vi "Configure Modulation (Pulse Width).vi"(0 "VISA resource name":refnum<visa-resource-name>, 1 "PWM Source (0: Internal)":i32(ring) items=["Internal", "External", "CH1", "CH2"], 2 "Internal Function (0: Sine)":i32(ring) items=["Sine", "Square", "RAMP", "NRAMP", "Triangle", "Noise", "PRBS", "Arbitrary"], 3 "PWM Deviation Duty Cycle (1 Percent)":dbl=1.0, 5 "Channel (1: 1)":i32(ring)=1 items=["1"=1, "2"=2], 7 "Enable Pulse Width Modulation(T: Enable)":bool=TRUE, 11 "error in (no error)":errorcluster, 12 "Deviation Setting Mode (0: Normal)":i32(ring) items=["Normal", "Duty Cycle"], 13 "PWM Internal Frequency/Sample Rate (10 Hz)":dbl=10.0, 14 "PWM Deviation (10 us)":dbl=1e-05) -> (4 "VISA resource name out":refnum<visa-resource-name>, 15 "error out":errorcluster)   [LabVIEW 2015, in "Agilent 3352X Series.lvlib"]
doc: "Allows and configures pulse width modulation. The width of a pulse waveform is varied by the instantaneous voltage of the modulating waveform.\n\n<b>Note</b>:\n(1) Before using this mode, all other modes must be turned off.\n(2) The carrier waveform must be Pulse.\n(3) The carrier waveform parameters are set by the Configure Pulse Waveform.vi"
uses:
  <instrlib>/Agilent 3352X Series/Agilent 3352X Series.lvlib
panel:
  # "Internal Pulse Width Modulation Settings"
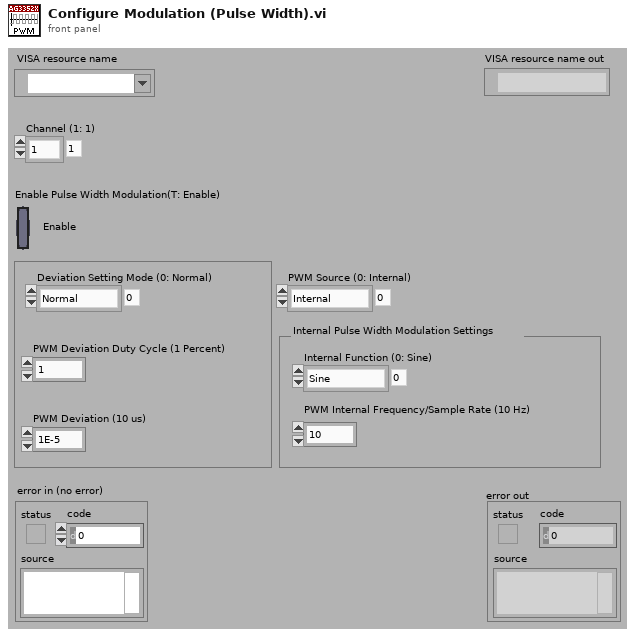
[diagram p1: front panel]
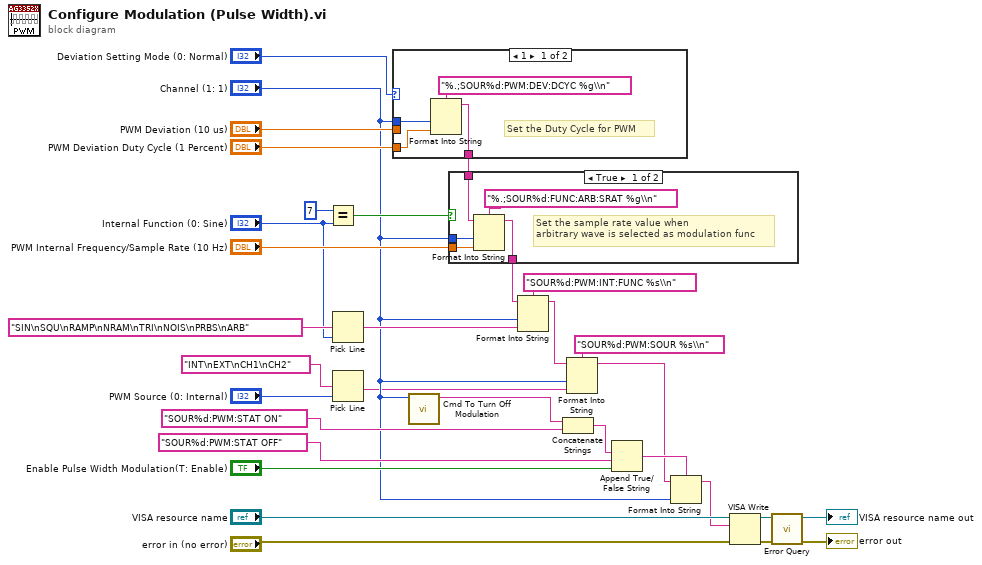
[diagram p0: block diagram]
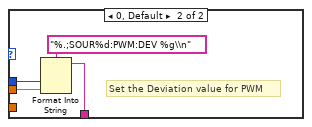
[diagram p2: hidden frame]
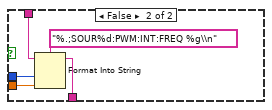
[diagram p3: hidden frame]
diagram:
  n1 = Equal?(x=u16 7, y="Internal Function (0: Sine)") -> (x = y?=w15:bool)
  n2 = Pick Line(multi-line string="SIN\nSQU\nRAMP\nNRAM\nTRI\nNOIS\nPRBS\nARB", line index="Internal Function (0: Sine)") -> (output string=w21:string)  [unwired: 1 out]
  n3 = Pick Line(multi-line string="INT\nEXT\nCH1\nCH2", line index="PWM Source (0: Internal)") -> (output string=w1:string)  [unwired: 1 out]
  n4 = case shown="1" "Deviation Setting Mode (0: Normal)" {
    tunnel: "Channel (1: 1)" -> [w35 w39]
    tunnel: "PWM Deviation (10 us)" -> [_ w38]
    tunnel: "PWM Deviation Duty Cycle (1 Percent)" -> [w34 _]
    tunnel: [w33 w37] -> w12
    frame 1 {
      # "Set the Duty Cycle for PWM"
      n5 = Format Into String(format string="%.;SOUR%d:PWM:DEV:DCYC %g\\n", w35, w34) -> (resulting string=w33:string)  [unwired: 2 in, 1 out]
    }
    frame 0, Default {
      # "Set the Deviation value for PWM"
      n6 = Format Into String(format string="%.;SOUR%d:PWM:DEV %g\\n", w39, w38) -> (resulting string=w37:string)  [unwired: 2 in, 1 out]
    }
  }
  n7 = call <instrlib>:"Cmd To Turn Off Modulation.vi"("Channel (1: 1)"="Channel (1: 1)") -> ("Cmd String"=w7:string)  [unwired: 10 out]
  n8 = case shown="True" w15 {
    tunnel: "Channel (1: 1)" -> [w43 w50]
    tunnel: w12 -> [w41 w49]
    tunnel: "PWM Internal Frequency/Sample Rate (10 Hz)" -> [w42 w47]
    tunnel: [w45 w46] -> w18
    frame True {
      # "Set the sample rate value when\narbitrary wave is selected as modulation func"
      n9 = Format Into String(format string="%.;SOUR%d:FUNC:ARB:SRAT %g\\n", initial string=w41, w43, w42) -> (resulting string=w45:string)  [unwired: 1 in, 1 out]
    }
    frame False {
      n10 = Format Into String(format string="%.;SOUR%d:PWM:INT:FREQ %g\\n", initial string=w49, w50, w47) -> (resulting string=w46:string)  [unwired: 1 in, 1 out]
    }
  }
  n11 = Format Into String(format string="SOUR%d:PWM:INT:FUNC %s\\n", initial string=w18, "Channel (1: 1)", w21) -> (resulting string=w31:string)  [unwired: 1 in, 1 out]
  n12 = Concatenate Strings(w7, "SOUR%d:PWM:STAT ON") -> (w10:string)
  n13 = Format Into String(format string="SOUR%d:PWM:SOUR %s\\n", initial string=w31, "Channel (1: 1)", w1) -> (resulting string=w2:string)  [unwired: 1 in, 1 out]
  n14 = Append True/False String(1:"Enable Pulse Width Modulation(T: Enable)", 2:"SOUR%d:PWM:STAT OFF", 3:w10) -> (0:w9:string)  [unwired: 1 out]
  n15 = Format Into String(format string=w9, initial string=w2, "Channel (1: 1)") -> (resulting string=w5:string)  [unwired: 1 in, 1 out]
  n16 = VISA Write(VISA resource name="VISA resource name", write buffer=w5, error in (no error)="error in (no error)") -> (VISA resource name out=w27:refnum<visa-resource-name>, error out=w26:errorcluster)  [unwired: 1 out]
  n17 = call <instrlib>:"Error Query.vi"("error in (no error)"=w26, "VISA resource name"=w27) -> ("error out"=→"error out":errorcluster, "VISA resource name out"=→"VISA resource name out":refnum<visa-resource-name>)  [unwired: 8 out]
